vi "BRig_RT_comm_webdav_upload_all__v3.vi"(0 "input_I_connected_webdav":bool, 1 "input_fileName_prefix":string, 5 "input_hSession":T1, 7 "input_error":errorcluster, 11 "input_True":bool) -> (6 "output_hSession":T1, 8 "error out":errorcluster, 12 "output_nFilenames":i32, 13 "output_arrFilenames":string[](array[string]), 14 "output_uploaded":bool[](array[boolean]), 15 "output_strCmd":string)   [LabVIEW 2014]
uses:
  <vilib>/WebDAVClient/Advanced/SessionHandle.ctl
  <vilib>/WebDAVClient/NI_WebDAV.lvlib
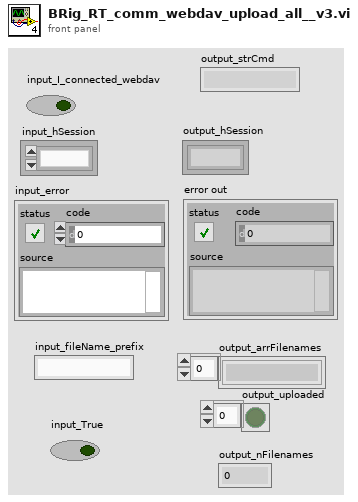
[diagram p1: front panel]
types:
  T1 = typedef "NI_WebDAV.lvlib/SessionHandle.ctl" = refnum<k1>
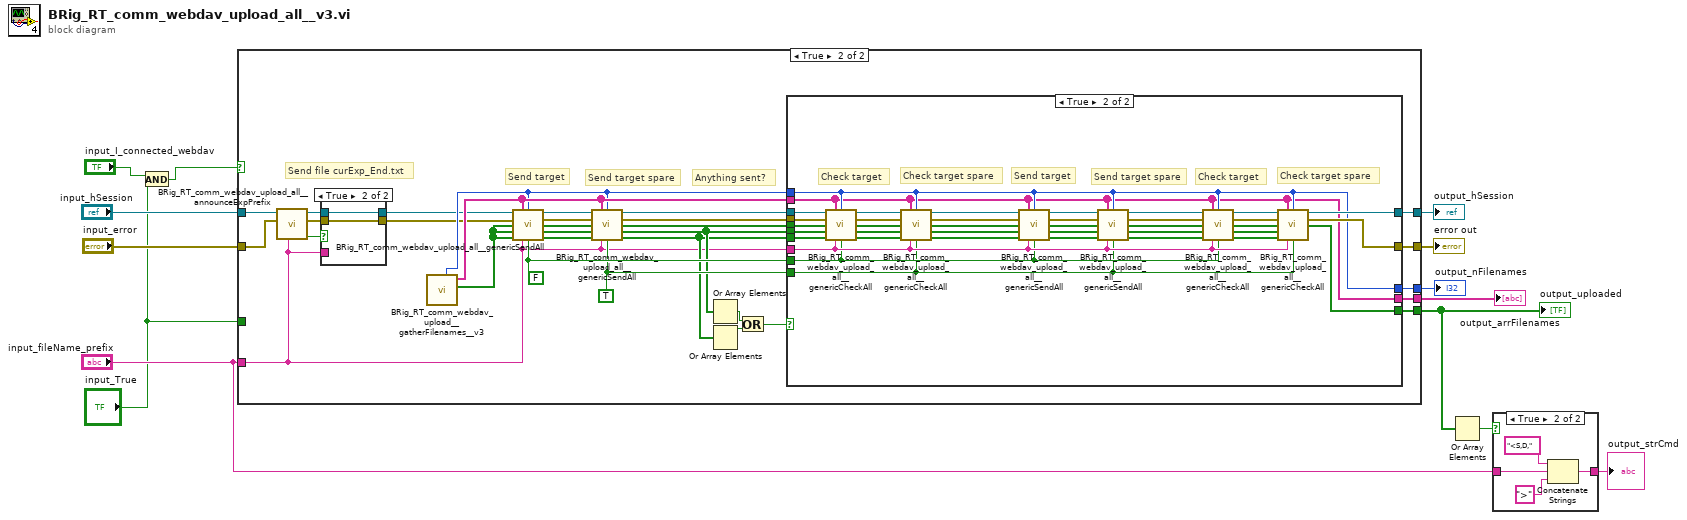
[diagram p0: block diagram]
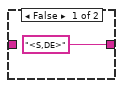
[diagram p2: hidden frame]
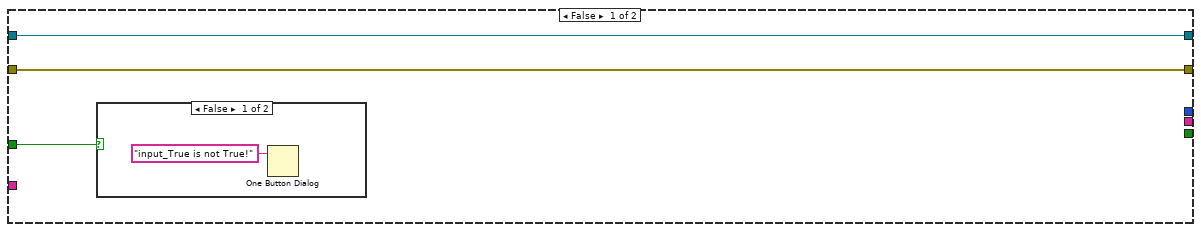
[diagram p3: hidden frame]
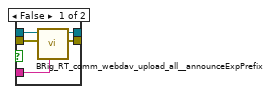
[diagram p5: hidden frame]
diagram:
  n1 = And(x="input_I_connected_webdav", y="input_True") -> (x .and. y?=w2:bool)
  n2 = case shown="True" w2 {
    tunnel: "input_hSession" -> [w16 w25]
    tunnel: [w16 w30] -> w12
    tunnel: "input_error" -> [w15 w24]
    tunnel: [w15 w29] -> w10
    tunnel: "input_fileName_prefix" -> [_ w20]
    tunnel: [_ w28] -> w8
    tunnel: [_ w27] -> w9
    tunnel: [_ w26] -> w7
    tunnel: "input_True" -> [w14 _]
    frame False {
      n3 = case shown="False" w14 {
        frame False {
          n4 = One Button Dialog(message="input_True is not True!") -> ()  [unwired: 1 in, 1 out]
        }
        frame True {
        }
      }
    }
    frame True {
      w38 = TRUE ("input_Target(F)_or_Spare(T)")
      w39 = FALSE ("input_Target(F)_or_Spare(T)")
      # "Send file curExp_End.txt"
      # "Anything sent?"
      # "Send target spare"
      # "Send target"
      n5 = call "BRig_RT_comm_webdav_upload_all__announceExpPrefix.vi"("input_fileName_prefix"=w20, "input_errro"=w24, "intput_hSession"=w25) -> ("output_checkData"=w21:bool, "output_error"=w22:errorcluster, "output_hSession"=w23:T1)  [unwired: 6 in]
      n6 = case shown="True" w21 {
        tunnel: w23 -> [w53 w55]
        tunnel: w22 -> [w52 w54]
        tunnel: w20 -> [w51 _]
        tunnel: [w50 w55] -> w19
        tunnel: [w49 w54] -> w18
        frame False {
          n7 = call "BRig_RT_comm_webdav_upload_all__announceExpPrefix.vi"("input_fileName_prefix"=w51, "input_errro"=w52, "intput_hSession"=w53) -> ("output_error"=w49:errorcluster, "output_hSession"=w50:T1)  [unwired: 6 in, 1 out]
        }
        frame True {
        }
      }
      n8 = call "BRig_RT_comm_webdav_upload__gatherFilenames__v3.vi"() -> ("output_arrBlank"=w48:bool[], "output_arrFilenames"=w37:string[], "output_n"=w36:i32)  [unwired: 9 in]
      n9 = call "BRig_RT_comm_webdav_upload_all__genericSendAll.vi"("input_hSession"=w19, "input_arrFilenames"=w37, "input_n"=w36, "input_error"=w18, "input_arrUploaded"=w48, "input_arrSentTarget"=w48, "input_arrSentTargetSpare"=w48, "input_fileName_prefix"=w20, "input_Target(F)_or_Spare(T)"=w39) -> ("output_hSession"=w47:T1, "output_error"=w46:errorcluster, "output_arrUploaded"=w45:bool[], "output_arrSentTarget"=w44:bool[], "output_arrSentTargetSpare"=w43:bool[])  [unwired: 2 in]
      n10 = call "BRig_RT_comm_webdav_upload_all__genericSendAll.vi"("input_hSession"=w47, "input_arrFilenames"=w37, "input_n"=w36, "input_error"=w46, "input_arrUploaded"=w45, "input_arrSentTarget"=w44, "input_arrSentTargetSpare"=w43, "input_fileName_prefix"=w20, "input_Target(F)_or_Spare(T)"=w38) -> ("output_hSession"=w42:T1, "output_error"=w41:errorcluster, "output_arrUploaded"=w40:bool[], "output_arrSentTarget"=w35:bool[], "output_arrSentTargetSpare"=w34:bool[])  [unwired: 2 in]
      n11 = Or Array Elements(Boolean array=w35) -> (logical OR=w32:bool)
      n12 = Or Array Elements(Boolean array=w34) -> (logical OR=w33:bool)
      n13 = Or(x=w32, y=w33) -> (x .or. y?=w31:bool)
      n14 = case shown="True" w31 {
        tunnel: w42 -> [w60 w98]
        tunnel: w41 -> [w59 w97]
        tunnel: w40 -> [w56 w96]
        tunnel: w39 -> [_ w67]
        tunnel: w20 -> [_ w68]
        tunnel: w38 -> [_ w66]
        tunnel: w37 -> [w57 w61]
        tunnel: w36 -> [w58 w62]
        tunnel: w35 -> [_ w90]
        tunnel: w34 -> [_ w89]
        tunnel: [w60 w65] -> w30
        tunnel: [w59 w64] -> w29
        tunnel: [w58 w62] -> w28
        tunnel: [w57 w61] -> w27
        tunnel: [w56 w63] -> w26
        frame False {
        }
        frame True {
          # "Check target spare"
          # "Check target"
          # "Send target spare"
          # "Send target"
          # "Check target spare"
          # "Check target"
          n15 = call "BRig_RT_comm_webdav_upload_all__genericCheckAll.vi"("input_hSession"=w98, "input_arrFilenames"=w61, "input_n"=w62, "input_error"=w97, "input_arrUploaded"=w96, "input_arrSentTarget"=w90, "input_arrSentTargetSpare"=w89, "input_fileName_prefix"=w68, "input_Target(F)_or_Spare(T)"=w67) -> ("output_hSession"=w95:T1, "output_error"=w94:errorcluster, "output_arrUploaded"=w93:bool[], "output_arrSentTarget"=w92:bool[], "output_arrSentTargetSpare"=w91:bool[])  [unwired: 2 in]
          n16 = call "BRig_RT_comm_webdav_upload_all__genericCheckAll.vi"("input_hSession"=w95, "input_arrFilenames"=w61, "input_n"=w62, "input_error"=w94, "input_arrUploaded"=w93, "input_arrSentTarget"=w92, "input_arrSentTargetSpare"=w91, "input_fileName_prefix"=w68, "input_Target(F)_or_Spare(T)"=w66) -> ("output_hSession"=w88:T1, "output_error"=w87:errorcluster, "output_arrUploaded"=w86:bool[], "output_arrSentTarget"=w85:bool[], "output_arrSentTargetSpare"=w84:bool[])  [unwired: 2 in]
          n17 = call "BRig_RT_comm_webdav_upload_all__genericSendAll.vi"("input_hSession"=w88, "input_arrFilenames"=w61, "input_n"=w62, "input_error"=w87, "input_arrUploaded"=w86, "input_arrSentTarget"=w85, "input_arrSentTargetSpare"=w84, "input_fileName_prefix"=w68, "input_Target(F)_or_Spare(T)"=w67) -> ("output_hSession"=w83:T1, "output_error"=w82:errorcluster, "output_arrUploaded"=w81:bool[], "output_arrSentTarget"=w80:bool[], "output_arrSentTargetSpare"=w79:bool[])  [unwired: 2 in]
          n18 = call "BRig_RT_comm_webdav_upload_all__genericSendAll.vi"("input_hSession"=w83, "input_arrFilenames"=w61, "input_n"=w62, "input_error"=w82, "input_arrUploaded"=w81, "input_arrSentTarget"=w80, "input_arrSentTargetSpare"=w79, "input_fileName_prefix"=w68, "input_Target(F)_or_Spare(T)"=w66) -> ("output_hSession"=w78:T1, "output_error"=w76:errorcluster, "output_arrUploaded"=w75:bool[], "output_arrSentTarget"=w74:bool[], "output_arrSentTargetSpare"=w73:bool[])  [unwired: 2 in]
          n19 = call "BRig_RT_comm_webdav_upload_all__genericCheckAll.vi"("input_hSession"=w78, "input_arrFilenames"=w61, "input_n"=w62, "input_error"=w76, "input_arrUploaded"=w75, "input_arrSentTarget"=w74, "input_arrSentTargetSpare"=w73, "input_fileName_prefix"=w68, "input_Target(F)_or_Spare(T)"=w67) -> ("output_hSession"=w77:T1, "output_error"=w72:errorcluster, "output_arrUploaded"=w71:bool[], "output_arrSentTarget"=w70:bool[], "output_arrSentTargetSpare"=w69:bool[])  [unwired: 2 in]
          n20 = call "BRig_RT_comm_webdav_upload_all__genericCheckAll.vi"("input_hSession"=w77, "input_arrFilenames"=w61, "input_n"=w62, "input_error"=w72, "input_arrUploaded"=w71, "input_arrSentTarget"=w70, "input_arrSentTargetSpare"=w69, "input_fileName_prefix"=w68, "input_Target(F)_or_Spare(T)"=w66) -> ("output_hSession"=w65:T1, "output_error"=w64:errorcluster, "output_arrUploaded"=w63:bool[])  [unwired: 2 in, 2 out]
        }
      }
    }
  }
  "error out" <- w10
  "output_hSession" <- w12
  "output_arrFilenames" <- w9
  "output_nFilenames" <- w8
  "output_uploaded" <- w7
  n21 = Or Array Elements(Boolean array=w7) -> (logical OR=w6:bool)
  n22 = case shown="True" w6 {
    tunnel: "input_fileName_prefix" -> [_ w101]
    tunnel: ["<S,DE>" ("string") w100] -> w4
    frame False {
    }
    frame True {
      n23 = Concatenate Strings("<S,D," ("string"), w101, ">" ("string")) -> (w100:string)
    }
  }
  "output_strCmd" <- w4
